vi "writeToXML.vi"(8 "error in (no error)":errorcluster, 10 "ClassLabel":string="TCSAtmosphericDispersionStatus", 11 "TCSAtmosphericDispersionStatus in":refnum<class "TCSAtmosphericDispersionStatus.lvclass">) -> (0 "error out":errorcluster, 2 "outputXMLString":string="<TCSAtmospericDispersionStatus>\n  <currentAtmosphericDispersion_arcsec>0</currentAtmosphericDispersion_arcsec>\n  <wavelength1>3E-7</wavelength1>\n  <wavelength2>6E-7</wavelength2>\n</TCSAtmospericDispersionStatus>", 3 "TCSAtmosphericDispersionStatus out":refnum<class "TCSAtmosphericDispersionStatus.lvclass">)   [LabVIEW 2014, in "TCSDataDefinitions.lvlib" / "TCSAtmosphericDispersionStatus.lvlib" / "TCSAtmosphericDispersionStatus.lvclass"]
uses:
  TCSAtmosphericDispersionStatus.lvclass
  <userlib>/Common/UnitsAndXML/FlattenItemWithUnitToXML/FlattenPlaneAngleToXML/PlaneAngleUnit.ctl
  <userlib>/Common/UnitsAndXML/FlattenItemWithUnitToXML/FlattenLengthToXML/LengthUnit.ctl
  TCSAtmosphericDispersionStatus.lvclass/TCSAtmosphericDispersionStatus.ctl
  <userlib>/Common/UnitsAndXML/UnitsAndXML.lvlib
  <userlib>/Common/XML/XMLGenerator/XMLGenerator.lvclass
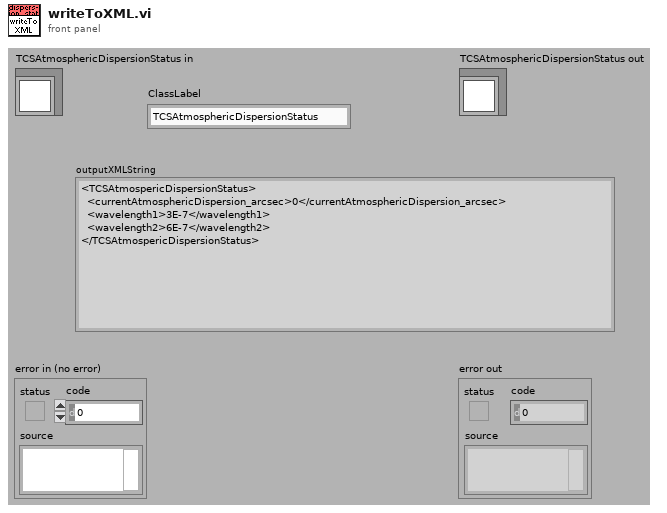
[diagram p1: front panel]
types:
  T1 = typedef "UnitsAndXML.lvlib/PlaneAngleUnit.ctl" = enum16{"rad", "deg", "'", "\""}
  T2 = typedef "UnitsAndXML.lvlib/LengthUnit.ctl" = enum16{"m", "Angstrom", "AU", "chain", "cm", "cubit", "fathom", "fermi", "ft", "furlong", "hubble", "in", "ly", "mi", "mm", "rod", "um", "yd"}
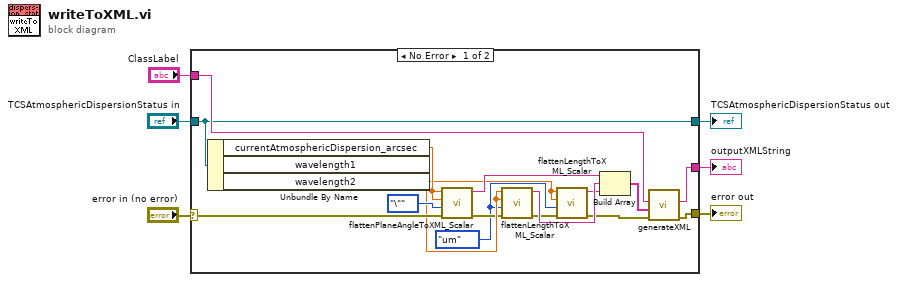
[diagram p0: block diagram]
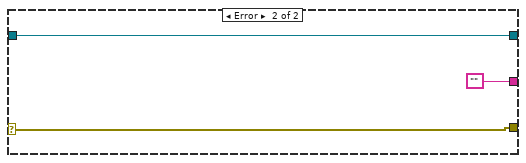
[diagram p2: hidden frame]
diagram:
  n1 = case shown="No Error" "error in (no error)" {
    selector: "error in (no error)" -> [w17 w26]
    tunnel: [w21 w26] -> w5
    tunnel: [w7 w25] -> w3
    tunnel: "TCSAtmosphericDispersionStatus in" -> [w7 w25]
    tunnel: [w20 ""] -> w2
    tunnel: "ClassLabel" -> [w23 _]
    frame No Error {
      w9 = LengthUnit."um" ("lengthUnitInXML")
      n2 = Unbundle By Name(w7) -> ("currentAtmosphericDispersion_arcsec"=w19:dbl[unit], "wavelength1"=w15:dbl[unit], "wavelength2"=w13:dbl[unit])
      n3 = call <userlib>:"flattenPlaneAngleToXML_Scalar.vi"("error in (no error)"=w17, "planeAngleUnitInXML"=PlaneAngleUnit."\"", "planeAngleAgain"=w19, "planeAngle"=w19) -> ("error out"=w14:errorcluster, "xmlString"=w16:string)  [unwired: 6 in]
      n4 = call <userlib>:"flattenLengthToXML_Scalar.vi"("error in (no error)"=w14, "lengthUnitInXML"=w9, "lengthAgain"=w15, "length"=w15) -> ("error out"=w11:errorcluster, "xmlString"=w12:string)  [unwired: 6 in]
      n5 = call <userlib>:"flattenLengthToXML_Scalar.vi"("error in (no error)"=w11, "lengthUnitInXML"=w9, "lengthAgain"=w13, "length"=w13) -> ("error out"=w10:errorcluster, "xmlString"=w8:string)  [unwired: 6 in]
      n6 = Build Array(w16, w12, w8) -> (w22:string[])
      n7 = call <userlib>:"generateXML.vi"("error in"=w10, "childrenXML"=w22, "elementName"=w23) -> ("error out"=w21:errorcluster, "XML out"=w20:string)  [unwired: 6 in, 1 out]
    }
    frame Error {
    }
  }
  "error out" <- w5
  "TCSAtmosphericDispersionStatus out" <- w3
  "outputXMLString" <- w2
